vi "2100_Read RFFE_w_Waveform_Publish Data.vi"(0 "Semiconductor Module Context":T2, 1 "Num_Reg_to_Read":u8=1, 2 "Published Data Id":string, 3 "Publish_Data?":bool, 5 "Pins":string[](array[string])=["CLK", "SDA"], 7 "Reg_Address_Data":T4={"Address"=81, "Data"=0} {"Address" format="%.0x"}, 9 "USID":T3 max=15, 11 "Error In":errorcluster, 12 "Bit_Location(LSB)":u8=7 max=7, 13 "#ofBits":u8=1 min=1 max=8) -> (4 "Ext_Read_Reg":i32[](array[numeric]), 6 "Ext_Read_Data":u8[](array[numeric])=[31, 144, 7], 8 "Converted Data":T5 {"Register" max=31 format="%.0x"; "Slave Address" max=15 format="%.0x"}, 10 "Reg Value":u8 format="%.0b", 15 "Error Out":errorcluster)   [LabVIEW 2013]
uses:
  <vilib>/NI_TestStand_SemiconductorModule/NI_TestStand_Semiconductor_Module.lvlibp/PinMap/General/SemiconductorModuleContext.ctl
  Controls/USID.ctl
  Controls/Reg_Address_Data.ctl
  MIPI_RFFE/Ctrls/RegReadWrite.ctl
  MIPI_RFFE/Ctrls/Configuration.ctl
  MIPI_RFFE/Ctrls/ClockDataChannels.ctl
  <vilib>/NI_TestStand_SemiconductorModule/NI_TestStand_Semiconductor_Module.lvlibp/PinMap/HSDIO/PinsToNIHSDIOSessions.vi
  <vilib>/Waveform/DWDTOps.llb/DWDT Digital Size.vi
  <instrlib>/niHSDIO/niHSDIO.llb/niHSDIO Write Named Waveform (WDT).vi
  <instrlib>/niHSDIO/niHSDIO.llb/niHSDIO Fetch Waveform (WDT).vi
  <vilib>/NI_TestStand_SemiconductorModule/NI_TestStand_Semiconductor_Module.lvlibp/PinMap/General/Publish/PublishDataDoubleFunctionalTest.vi
  <vilib>/NI_TestStand_SemiconductorModule/NI_TestStand_Semiconductor_Module.lvlibp
panel:
  in  "Tab Control":T1(tab)
  out "Waveform Graph":digitalwaveform(graph)
  # "Specific Bits"
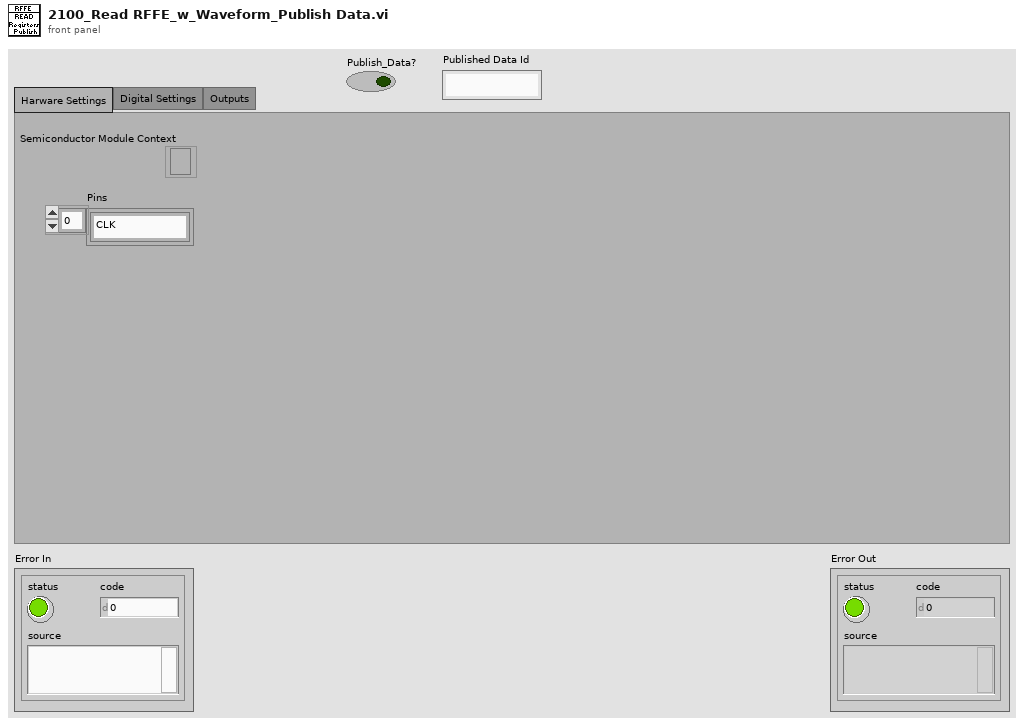
[diagram p1: front panel]
types:
  T1 = enum32{"Harware Settings", "Digital Settings", "Outputs"}
  T2 = typedef "NI_TestStand_Semiconductor_Module.lvlibp/SemiconductorModuleContext.ctl" = refnum<k7>
  T3 = typedef "USID.ctl" = u8
  T4 = typedef "Reg_Address_Data.ctl" = cluster{"Address":u8, "Data":u8}
  T5 = cluster{"Slave Address":u8, "Register":u8, "Data":u8}
  T6 = typedef "Configuration.ctl" = cluster{"Samples to Allocate":i32, "Oversample Factor":u8, "Clock Channel":T7, "Data Channel":T7}
  T7 = typedef "ClockDataChannels.ctl" = enum16{"0", "1"}
  T8 = typedef "RegReadWrite.ctl" = cluster{"Slave Address":u8, "Register":u8, "Data":u8, "SetID_Pin_State":enum16{"0", "1", "Z"}}
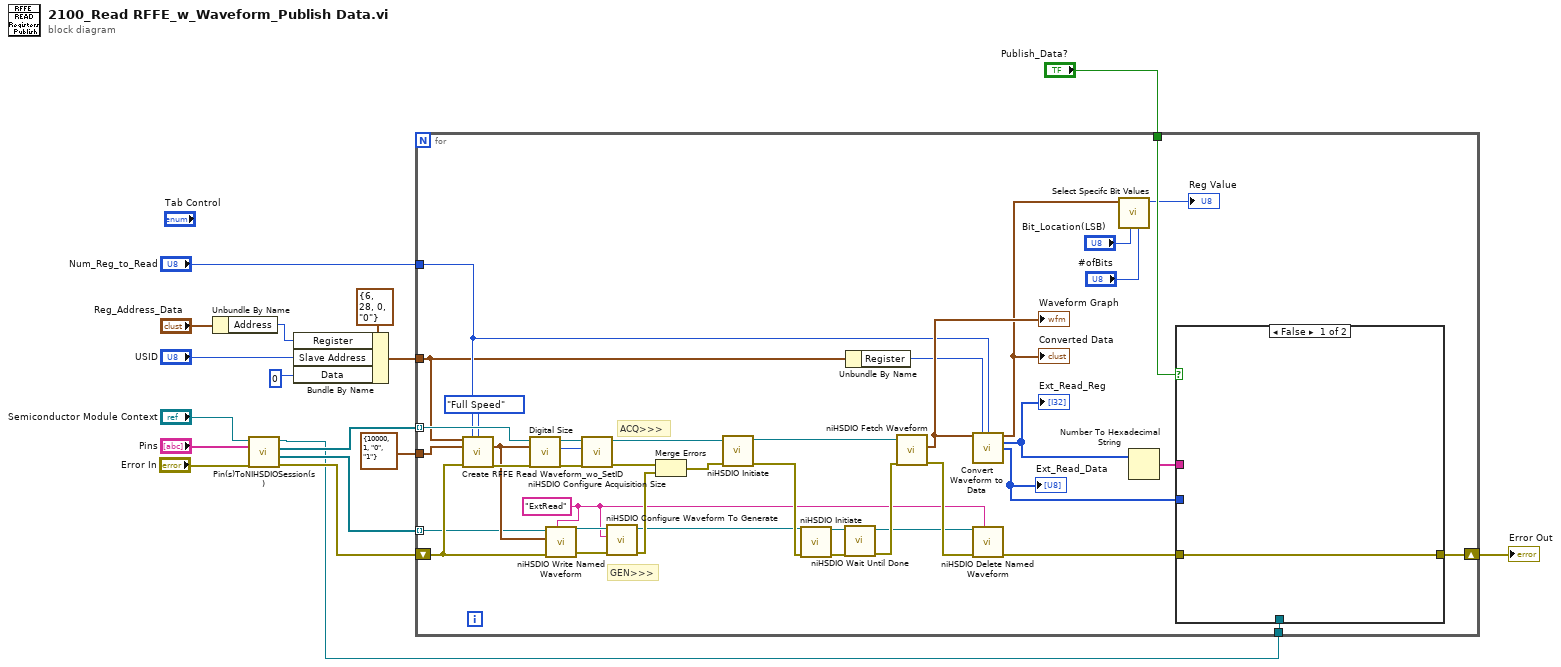
[diagram p0: block diagram]
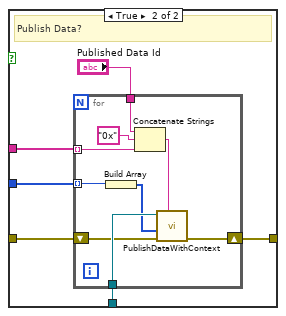
[diagram p2: hidden frame]
diagram:
  n1 = Unbundle By Name("Reg_Address_Data") -> ("Address"=w4:u8)
  n2 = call-poly <vilib>:"Pin(s)ToNIHSDIOSession(s).vi"("error in (no error)"="Error In", "Pins"="Pins", "Semiconductor Module Context"="Semiconductor Module Context") -> ("error out"=w15:errorcluster, "Generation Sessions"=w16:refnum<k15>[], "Acquisition Sessions"=w17:refnum<k15>[], "Semiconductor Module Context Out"=w6:T2)  [unwired: 3 in, 2 out]
  n3 = Bundle By Name(cluster=T8 {"Slave Address"=6, "Register"=28, "Data"=0, "SetID_Pin_State"=enum."0"} ("Data"), "Register"=w4, "Slave Address"="USID", "Data"=u8 0) -> (w10:T8)
  n4 = for {
    tunnel: w17 -> [w49] mode=indexing
    tunnel: w16 -> [w24] mode=indexing
    tunnel: w10 -> [w32]
    tunnel: T6 {"Samples to Allocate"=10000, "Oversample Factor"=1, "Clock Channel"=enum."0", "Data Channel"=enum."1"} ("Configuratation") -> [w47]
    shift-right: [w30] -> w1
    shift-left: w15 -> [w25]
    tunnel: "Num_Reg_to_Read" -> [w33]
    tunnel: w6 -> [w26]
    tunnel: "Publish_Data?" -> [w22]
    w36 = "ExtRead" ("waveform name (default:\"\")")
    # "GEN>>>"
    # "ACQ>>>"
    n5 = call "Create RFFE Read Waveform_wo_SetID.vi"("Data"=w32, "Ext_Read_Num_Reg"=w33, "Readback Speed"=enum16{"Full Speed", "Half Speed"}."Full Speed", "Configuratation"=w47, "error in (no error)"=w25) -> ("Waveform Graph"=w34:digitalwaveform, "error out"=w50:errorcluster)  [unwired: 9 in]
    n6 = call-poly <vilib>:"Digital Size.vi"("error in (no error)"=w50, "digital waveform in"=w34) -> ("error out"=w51:errorcluster, "number of samples"=w52:i32)  [unwired: 6 in, 2 out]
    n7 = call-poly <instrlib>:"niHSDIO Write Named Waveform.vi"("waveform name (default:\"\")"=w36, "error in (no error)"=w25, "data"=w34, "instrument handle"=w24) -> ("error out"=w42:errorcluster, "instrument handle out"=w40:refnum<k15>)  [unwired: 6 in]
    n8 = call <instrlib>:"niHSDIO Configure Acquisition Size.vi"("error in (no error)"=w51, "samples per record (1000 samples)"=w52, "instrument handle"=w49) -> ("error out"=w48:errorcluster, "instrument handle out"=w53:refnum<k15>)  [unwired: 7 in]
    n9 = call <instrlib>:"niHSDIO Configure Waveform To Generate.vi"("error in (no error)"=w42, "waveform name"=w36, "instrument handle"=w40) -> ("error out"=w41:errorcluster, "instrument handle out"=w39:refnum<k15>)  [unwired: 7 in]
    n10 = Merge Errors(w48, w41) -> (w54:errorcluster)
    n11 = call <instrlib>:"niHSDIO Initiate.vi"("error in (no error)"=w54, "instrument handle"=w53) -> ("error out"=w56:errorcluster, "instrument handle out"=w43:refnum<k15>)  [unwired: 8 in]
    n12 = call <instrlib>:"niHSDIO Initiate.vi"("error in (no error)"=w56, "instrument handle"=w39) -> ("error out"=w55:errorcluster, "instrument handle out"=w44:refnum<k15>)  [unwired: 8 in]
    n13 = call <instrlib>:"niHSDIO Wait Until Done.vi"("error in (no error)"=w55, "instrument handle"=w44) -> ("error out"=w46:errorcluster, "instrument handle out"=w37:refnum<k15>)  [unwired: 8 in]
    n14 = Unbundle By Name(w32) -> ("Register"=w31:u8)
    n15 = call-poly <instrlib>:"niHSDIO Fetch Waveform.vi"("error in (no error)"=w46, "instrument handle"=w43) -> ("error out"=w38:errorcluster, "data"=w35:digitalwaveform)  [unwired: 6 in, 2 out]
    "Waveform Graph" <- w35
    n16 = call "Convert Waveform to Data.vi"("Waveform Graph"=w35, "Register"=w31, "Ext_Read_Num_Reg"=w33) -> ("Converted Data"=w21:T5, "Ext_Read_Reg"=w28:i32[], "Ext_Read_Data"=w29:u8[])  [unwired: 10 in]
    "Converted Data" <- w21
    "Ext_Read_Reg" <- w28
    "Ext_Read_Data" <- w29
    n17 = call <instrlib>:"niHSDIO Delete Named Waveform.vi"("waveform name (default:\"\")"=w36, "error in (no error)"=w38, "instrument handle"=w37) -> ("error out"=w23:errorcluster)  [unwired: 7 in, 1 out]
    n18 = call "Select Specifc Bit Values.vi"("#ofBits"="#ofBits", "Bit_Location(LSB)"="Bit_Location(LSB)", "Converted Data"=w21) -> ("Bits"=→"Reg Value":u8)  [unwired: 8 in]
    n19 = Number To Hexadecimal String(2:w28) -> (0:w27:string[])  [unwired: 1 in]
    n20 = case shown="False" w22 {
      tunnel: [w57 w63] -> w30
      tunnel: w29 -> [_ w62]
      tunnel: w27 -> [_ w61]
      tunnel: w26 -> [_ w60]
      tunnel: w23 -> [w57 w59]
      frame False {
      }
      frame True {
        # "Publish Data?"
        n21 = for {
          tunnel: w60 -> [w71]
          tunnel: "Published Data Id" -> [w70]
          tunnel: w61 -> [w65] mode=indexing
          tunnel: w62 -> [w67] mode=indexing
          shift-right: [w72] -> w63
          shift-left: w59 -> [w64]
          n22 = Build Array(w67) -> (w66:u8[])
          n23 = Concatenate Strings(w70, "0x" ("string"), w65) -> (w68:string)
          n24 = call-poly <vilib>:"PublishDataWithContext.vi"("Published Data Id"=w68, "error in (no error)"=w64, "Data In"=w66, "Semiconductor Module Context"=w71) -> ("error out"=w72:errorcluster)  [unwired: 6 in, 1 out]
        }
      }
    }
  }
  "Error Out" <- w1
